vi "Video read with led for 2 part.vi"() -> ()   [LabVIEW 2009]
uses:
  <vilib>/vision/Image Controls.llb/IMAQ Image.ctl
  <vilib>/Instr/_visa.llb/VISA Configure Serial Port (Instr).vi
  <vilib>/Analysis/3filter.llb/Filter Passband Type.ctl
  <vilib>/Analysis/3filter.llb/Butterworth Filter (DBL).vi
  <vilib>/vision/NI_Vision_Development_Module.lvlib
  <vilib>/Analysis/NI_AALBase.lvlib
panel:
  out "cluster":T1
  in  "baud rate (9600)":u32=9600
  in  "VISA resource name":refnum<visa-resource-name>
  out "number":u32
  out "decimal integer string":string
  out "Image Dst Out":T2
  out "Blue Line":T3={"Global Rectangle"=[243, 262, 261, 384], "Contours"=[{"ID"=enum."External", "Type"=2, "Coordinates"=[260, 383, 243, 262]}]} {"Contours"."Type" items=["No Selection", "Point", "Line", "Rectangle", "Oval", "Polygon", "Freehand Region", "Annulus", "Unused2", "Unused3", "Broken Line", "Freehand Line", "Rotated Rectangle"]}
  out "Red Line":T3={"Global Rectangle"=[168, 264, 180, 378], "Contours"=[{"ID"=enum."External", "Type"=2, "Coordinates"=[168, 377, 179, 264]}]} {"Contours"."Type" items=["No Selection", "Point", "Line", "Rectangle", "Oval", "Polygon", "Freehand Region", "Annulus", "Unused2", "Unused3", "Broken Line", "Freehand Line", "Rotated Rectangle"]}
  in  "low  2":dbl=0.12500000000000006 format="%0.4f"
  in  "high 2":dbl=60.0 format="%0.2f"
  in  "sampling 2":dbl=1.0 format="%0.2f"
  out "LED BLUE":bool
  out "Waveform BLUE":dbl[](graph)
  in  "playtime":dbl=30.0
  out "Frame Number":i32
  in  "Frame Start":i32=2400
  out "LED RED":bool
  in  "low":dbl=0.12500000000000006 format="%0.4f"
  out "Waveform RED":dbl[](graph)
  in  "high":dbl=60.0 format="%0.2f"
  in  "sampling":dbl=1.0 format="%0.2f"
  out "Image":T2(plugin-control)
  in  "stop":bool
  in  "AVI Path":path
  # "RED"
  # "BLUE"
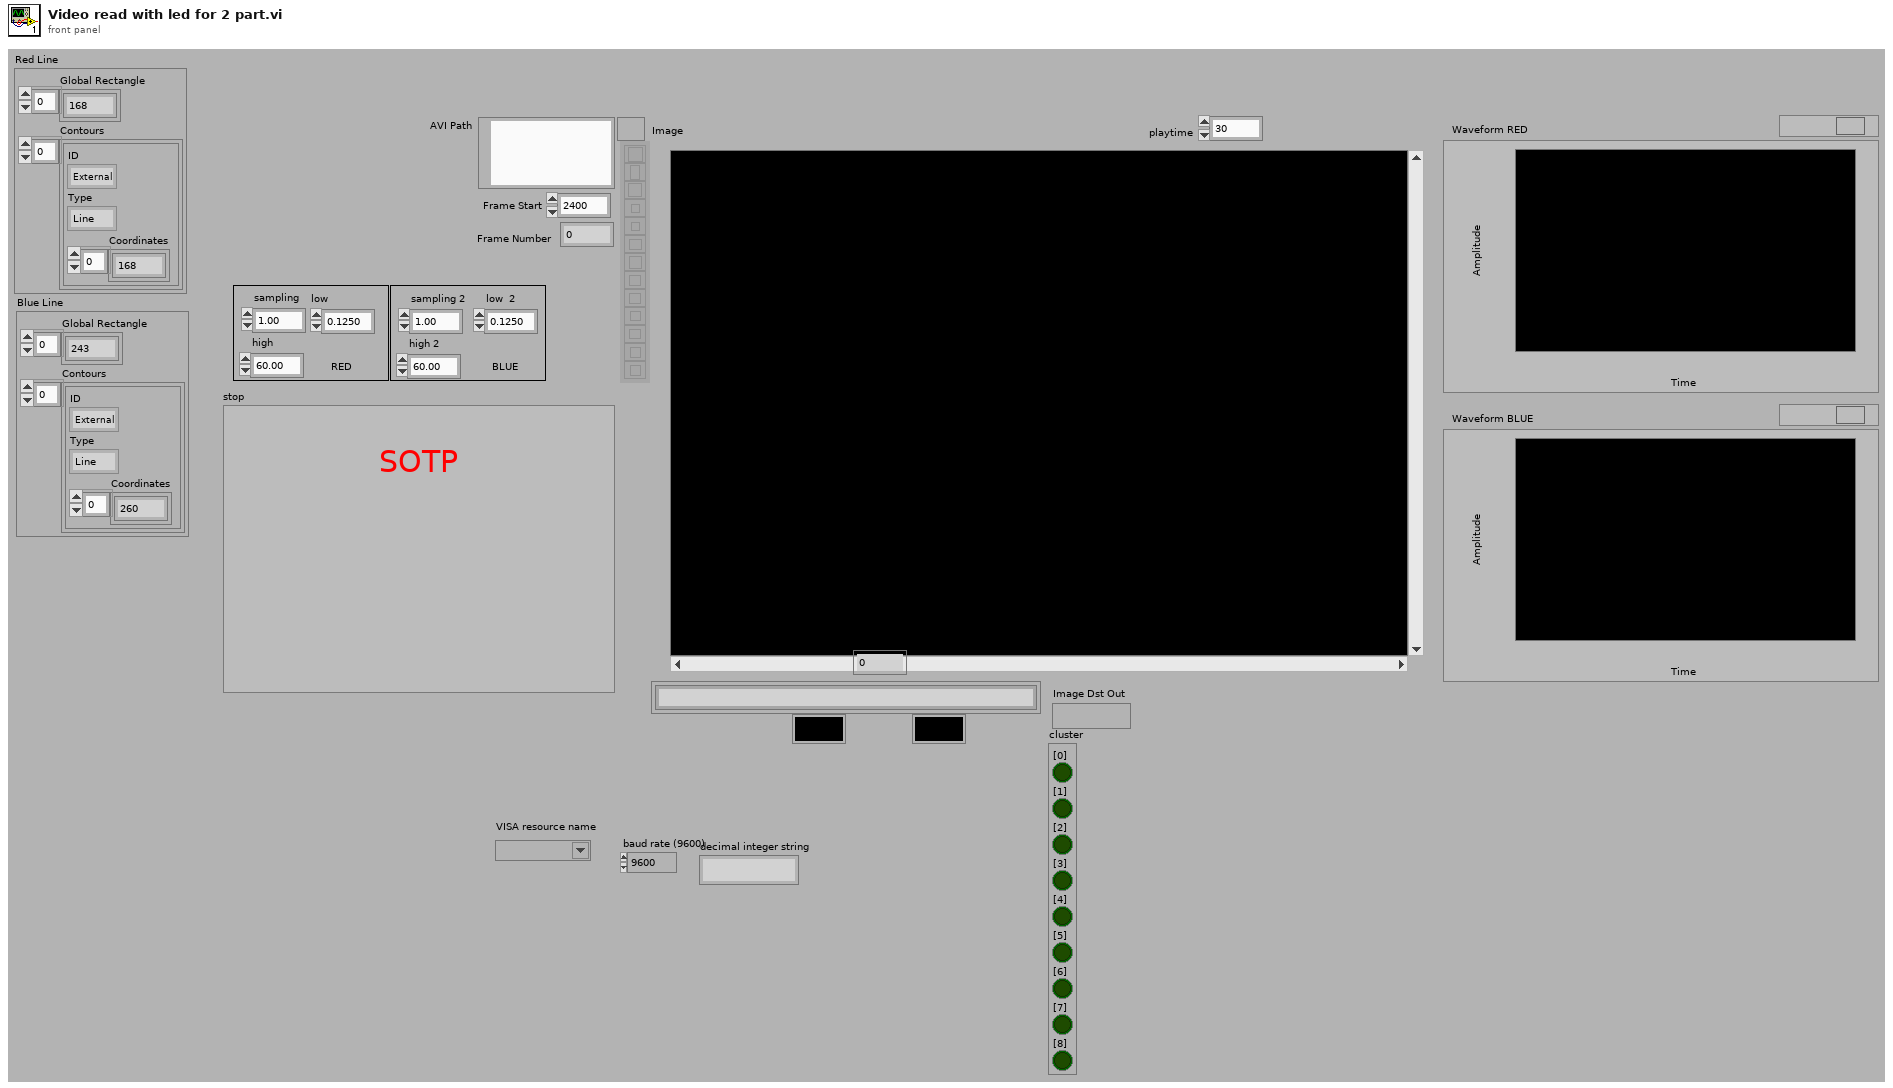
[diagram p1: front panel]
types:
  T1 = cluster{"[0]":bool, "[1]":bool, "[2]":bool, "[3]":bool, "[4]":bool, "[5]":bool, "[6]":bool, "[7]":bool, "[8]":bool}
  T2 = typedef "IMAQ Image.ctl" = refnum<image>
  T3 = cluster{"Global Rectangle":i32[], "Contours":cluster{"ID":enum32{"External", "Internal"}, "Type":u32, "Coordinates":i32[]}[]}
  T4 = typedef "NI_AALBase.lvlib/Filter Passband Type.ctl" = enum32{"Lowpass", "Highpass", "Bandpass", "Bandstop"}
  T5 = cluster{"Left":i32, "Top":i32, "Right":i32, "Bottom":i32}
  T6 = typedef "Image Type" = u32
  T7 = typedef "AviRefnum.ctl" = refnum<k1>
  T8 = cluster{"ID":enum32{"External", "Internal"}, "Type":u32, "Coordinates":i32[]}[]
  T9 = cluster{"ID":enum32{"External", "Internal"}, "Type":u32, "Coordinates":i32[]}
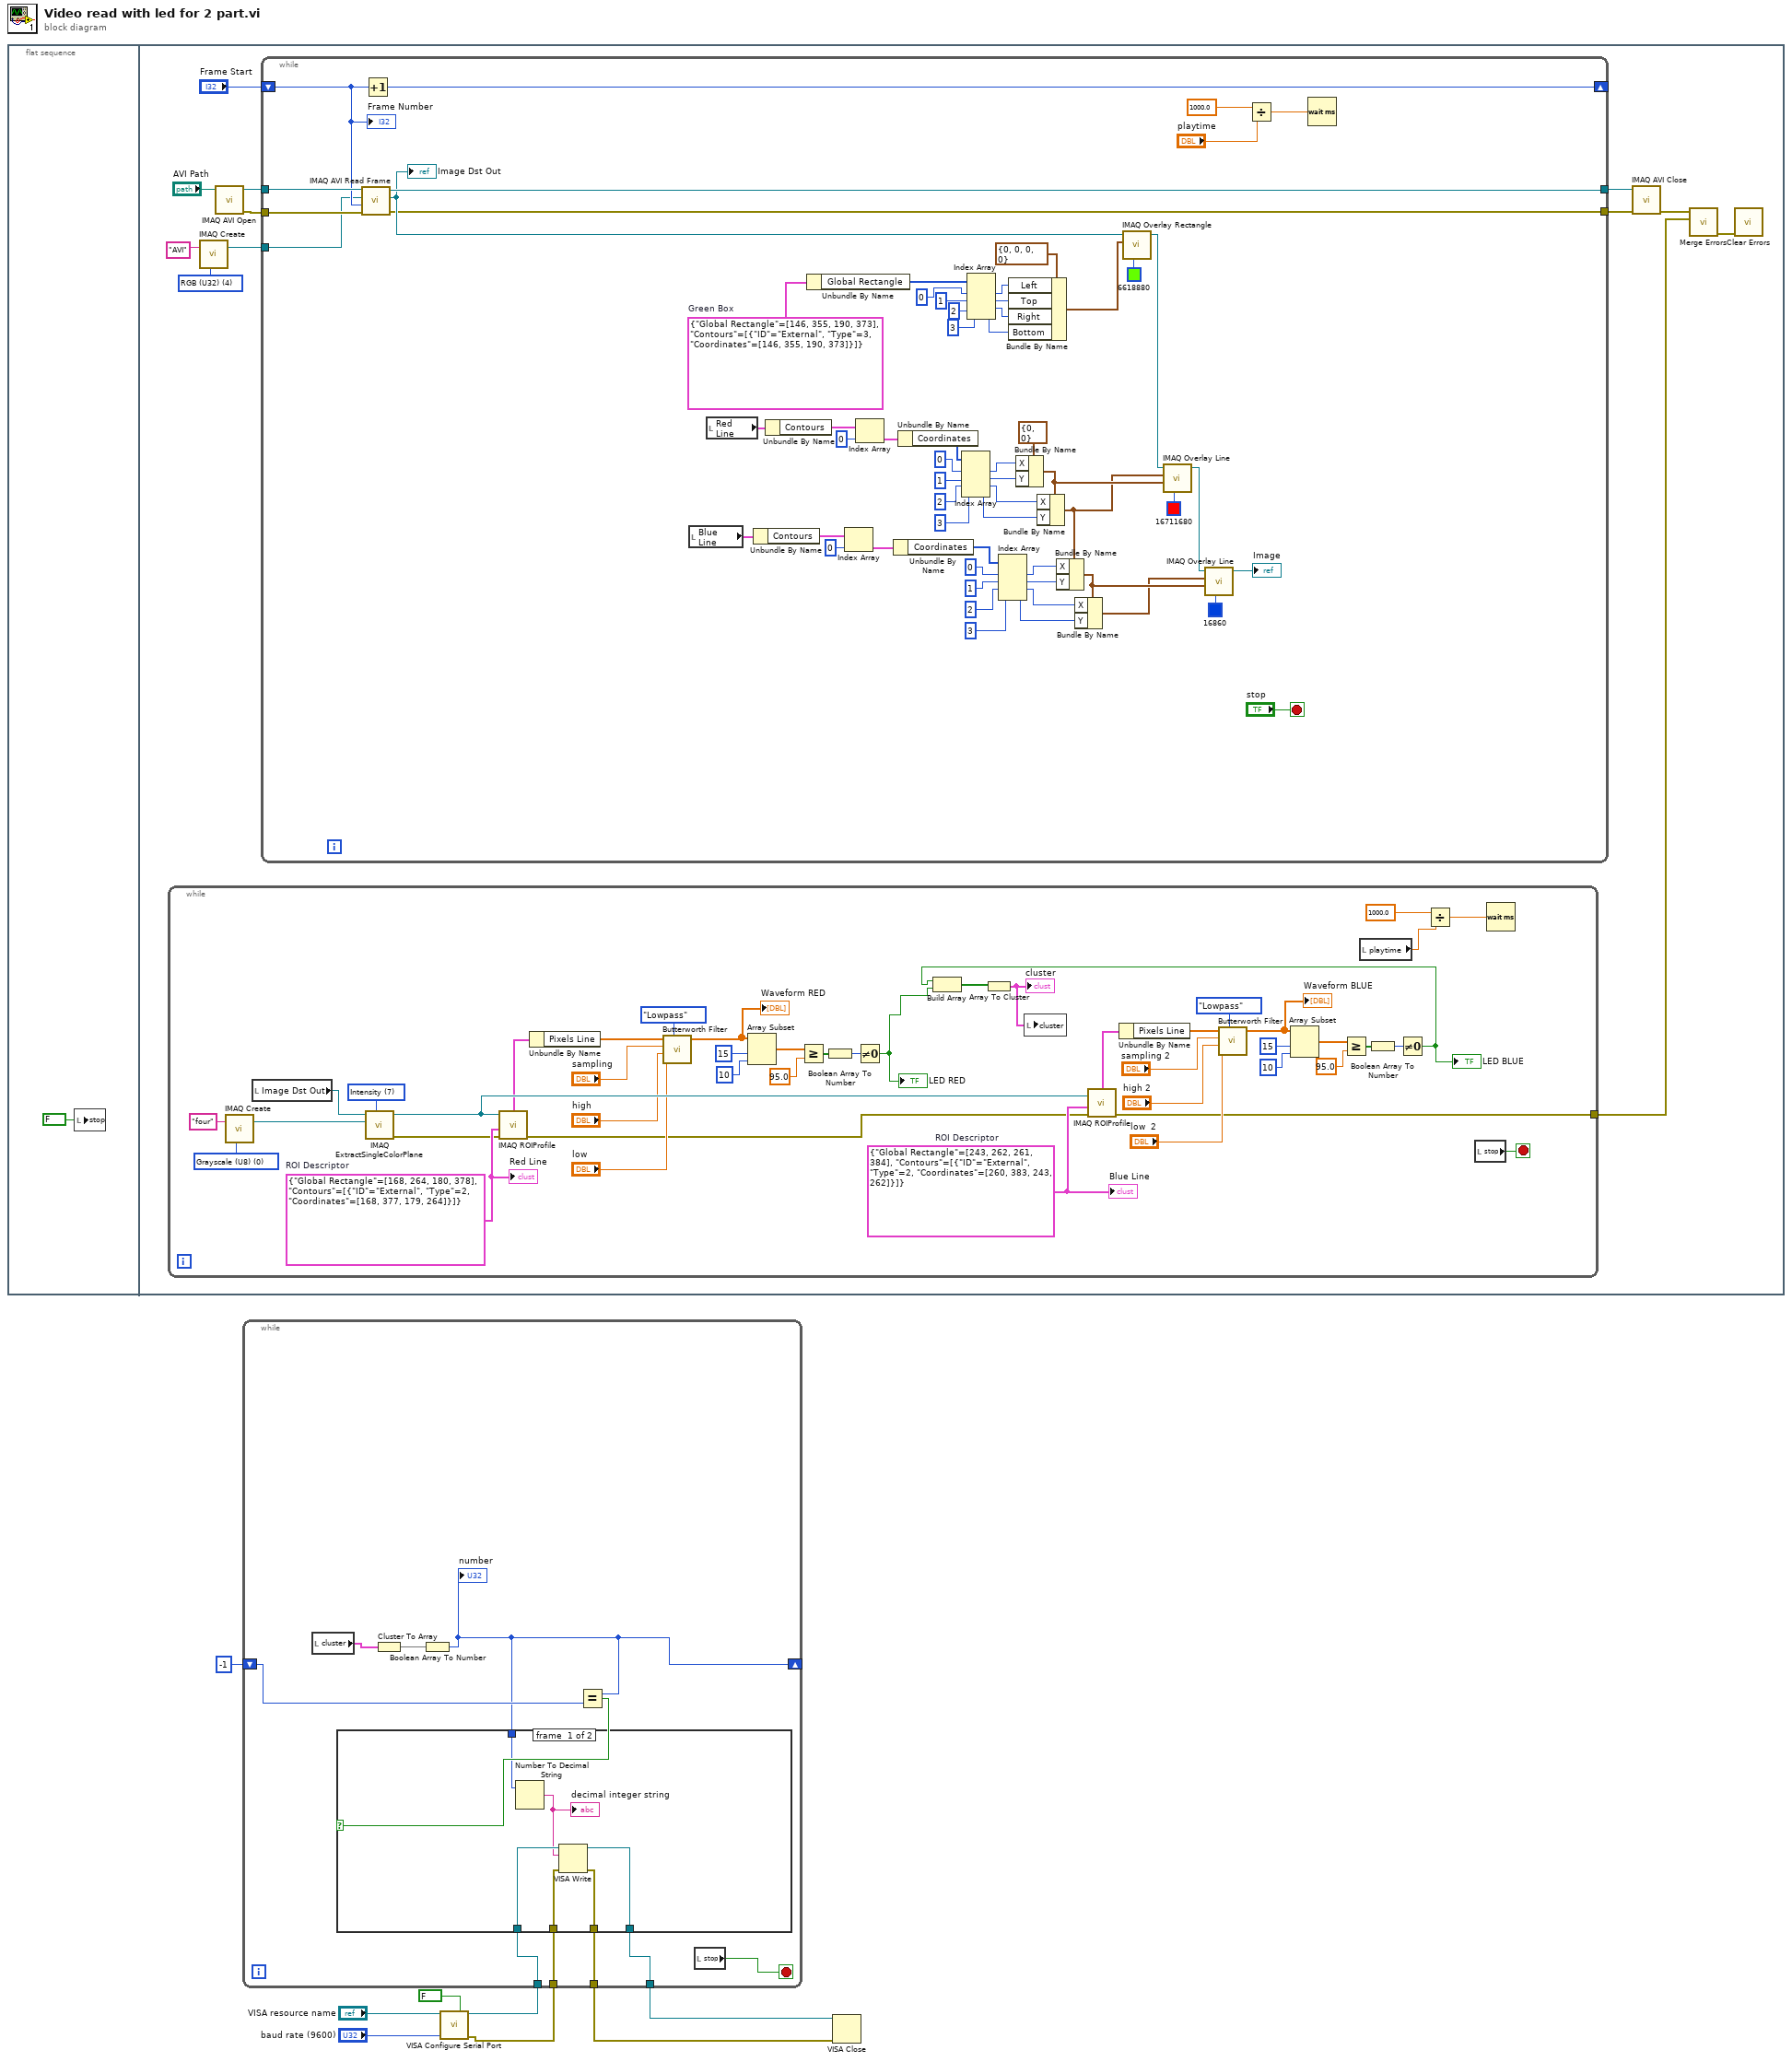
[diagram p0: block diagram]
diagram:
  n1 = flat-sequence {
    frame #0 {
      n2 = local write "stop"(FALSE ("stop")) -> ()
    }
    frame #1 {
      w12 = T6 4 items=["Grayscale (U8)", "Grayscale (I16)", "Grayscale (SGL)", "Complex (CSG)", "RGB (U32)", "HSL (U32)", "RGB (U64)", "Grayscale (U16)"] ("Image Type")
      n3 = while {
        tunnel: [w29] -> w15
        stop <- w64 stop-if-true
        w28 = T6 0 items=["Grayscale (U8)", "Grayscale (I16)", "Grayscale (SGL)", "Complex (CSG)", "RGB (U32)", "HSL (U32)", "RGB (U64)", "Grayscale (U16)"] ("Image Type")
        w62 = T3 {"Global Rectangle"=[243, 262, 261, 384], "Contours"=[{"ID"=enum."External", "Type"=2, "Coordinates"=[260, 383, 243, 262]}]}  # ROI Descriptor
        w63 = T3 {"Global Rectangle"=[168, 264, 180, 378], "Contours"=[{"ID"=enum."External", "Type"=2, "Coordinates"=[168, 377, 179, 264]}]}  # ROI Descriptor
        w66 = 7 items=["Red", "Green", "Blue", "Hue", "Saturation", "Luminance", "Value", "Intensity"] ("Color Plane")
        n4 = call "IMAQ Create"("Image Name"="four", "Image Type"=w28) -> ("New Image"=w26:T2)  [unwired: 3 in, 1 out]
        n5 = local read "Image Dst Out"() -> (w31:T2)
        n6 = call "IMAQ ExtractSingleColorPlane"("Color Plane"=w66, "Image Dst"=w26, "Image Src"=w31) -> ("error out"=w30:errorcluster, "Image Dst Out"=w65:T2)  [unwired: 1 in, 6 out]
        n7 = call "IMAQ ROIProfile"("error in (no error)"=w30, "ROI Descriptor"=w63, "Image"=w65) -> ("error out"=w32:errorcluster, "ROI Graph"=w60:cluster{"x0":sgl, "dx":sgl, "Pixels Line":sgl[]})  [unwired: 4 out]
        n8 = Unbundle By Name(w60) -> ("Pixels Line"=w59:sgl[])
        n9 = call-poly <vilib>:"Butterworth Filter.vi"("filter type"=Filter_Passband_Type."Lowpass", "low cutoff freq: fl"="low", "high cutoff freq: fh"="high", "sampling freq: fs"="sampling", "X"=w59) -> ("Filtered X"=w55:dbl[])  [unwired: 3 in, 1 out]
        "Waveform RED" <- w55
        n10 = Array Subset(array=w55, index=15, length=10) -> (w52:dbl[])
        n11 = Greater Or Equal?(x=w52, y=95.0) -> (x >= y?=w50:bool[])
        n12 = Boolean Array To Number(Boolean array=w50) -> (number=w47:u32)
        n13 = Not Equal To 0?(x=w47) -> (x != 0?=w22:bool)
        "LED RED" <- w22
        n14 = call "IMAQ ROIProfile"("error in (no error)"=w32, "ROI Descriptor"=w62, "Image"=w65) -> ("error out"=w29:errorcluster, "ROI Graph"=w35:cluster{"x0":sgl, "dx":sgl, "Pixels Line":sgl[]})  [unwired: 4 out]
        n15 = Unbundle By Name(w35) -> ("Pixels Line"=w38:sgl[])
        n16 = call-poly <vilib>:"Butterworth Filter.vi"("filter type"=Filter_Passband_Type."Lowpass", "low cutoff freq: fl"="low  2", "high cutoff freq: fh"="high 2", "sampling freq: fs"="sampling 2", "X"=w38) -> ("Filtered X"=w34:dbl[])  [unwired: 3 in, 1 out]
        "Waveform BLUE" <- w34
        n17 = Array Subset(array=w34, index=15, length=10) -> (w43:dbl[])
        n18 = Greater Or Equal?(x=w43, y=95.0) -> (x >= y?=w41:bool[])
        n19 = local read "playtime"() -> (w46:dbl)
        n20 = Boolean Array To Number(Boolean array=w41) -> (number=w40:u32)
        n21 = Not Equal To 0?(x=w40) -> (x != 0?=w23:bool)
        "LED BLUE" <- w23
        n22 = Build Array(w23, w22) -> (w25:bool[])
        n23 = Array To Cluster(array=w25) -> (cluster=w24:T1)
        "cluster" <- w24
        n24 = local write "cluster"(w24) -> ()
        n25 = Divide(x=1000.0, y=w46) -> (x/y=w49:dbl)
        n26 = local read "stop"() -> (w64:bool)
        n27 = Wait (ms)(milliseconds to wait=w49) -> ()  [unwired: 1 out]
        "Red Line" <- w63
        "Blue Line" <- w62
      }
      n28 = call "IMAQ Create"("Image Name"="AVI", "Image Type"=w12) -> ("New Image"=w10:T2)  [unwired: 3 in, 1 out]
      n29 = call "IMAQ AVI Open"("AVI Path"="AVI Path") -> ("error out"=w18:errorcluster, "Avi Refnum"=w19:T7)  [unwired: 9 in]
      n30 = while {
        tunnel: w19 -> [w127]
        tunnel: w18 -> [w72]
        tunnel: [w126] -> w20
        shift-right: [w121] -> _
        shift-left: "Frame Start" -> [w120]
        tunnel: [w68] -> w13
        tunnel: w10 -> [w67]
        stop <- "stop" stop-if-true
        w119 = T3 {"Global Rectangle"=[146, 355, 190, 373], "Contours"=[{"ID"=enum."External", "Type"=3, "Coordinates"=[146, 355, 190, 373]}]}  # Green Box
        n31 = call "IMAQ AVI Read Frame"("error in (no error)"=w72, "Frame Number"=w120, "Image"=w67, "Avi Refnum"=w127) -> ("error out"=w68:errorcluster, "Image Out"=w69:T2, "Avi Refnum (duplicate)"=w126:T7)  [unwired: 4 in, 1 out]
        "Image Dst Out" <- w69
        n32 = Increment(x=w120) -> (x+1=w121:i32)
        n33 = local read "Blue Line"() -> (w71:T3)
        n34 = local read "Red Line"() -> (w70:T3)
        n35 = Unbundle By Name(w71) -> ("Contours"=w86:T8)
        n36 = Unbundle By Name(w70) -> ("Contours"=w101:T8)
        n37 = Unbundle By Name(w119) -> ("Global Rectangle"=w115:i32[])
        n38 = Index Array(array=w86, index=0) -> (element=w85:T9)
        n39 = Index Array(array=w101, index=0) -> (element=w103:T9)
        n40 = Unbundle By Name(w85) -> ("Coordinates"=w84:i32[])
        n41 = Unbundle By Name(w103) -> ("Coordinates"=w104:i32[])
        n42 = Index Array(array=w104, index #1=0 ("index"), index #2=1 ("index"), index #3=2 ("index"), index #4=3 ("index")) -> (element #1=w96:i32, element #2=w97:i32, element #3=w98:i32, element #4=w99:i32)
        n43 = Index Array(array=w115, index #1=0 ("index"), index #2=1 ("index"), index #3=2 ("index"), index #4=3 ("index")) -> (element #1=w114:i32, element #2=w113:i32, element #3=w112:i32, element #4=w111:i32)
        n44 = Index Array(array=w84, index #1=0 ("index"), index #2=1 ("index"), index #3=2 ("index"), index #4=3 ("index")) -> (element #1=w83:i32, element #2=w89:i32, element #3=w88:i32, element #4=w87:i32)
        n45 = Bundle By Name(cluster=T5 {"Left"=0, "Top"=0, "Right"=0, "Bottom"=0} ("Rectangle"), "Left"=w114, "Top"=w113, "Right"=w112, "Bottom"=w111) -> (w117:T5)
        n46 = Bundle By Name(cluster=cluster{"X":i32, "Y":i32} {"X"=0, "Y"=0} ("End Point"), "X"=w96, "Y"=w97) -> (w105:cluster{"X":i32, "Y":i32})
        n47 = Bundle By Name(cluster=w105, "X"=w98, "Y"=w99) -> (w75:cluster{"X":i32, "Y":i32})
        n48 = Bundle By Name(cluster=w75, "X"=w83, "Y"=w89) -> (w90:cluster{"X":i32, "Y":i32})
        n49 = Bundle By Name(cluster=w90, "X"=w88, "Y"=w87) -> (w81:cluster{"X":i32, "Y":i32})
        n50 = call "IMAQ Overlay Rectangle"("Color"=u32 6618880, "Rectangle"=w117, "Image"=w69) -> ("Image Out"=w91:T2)  [unwired: 7 in, 1 out]
        n51 = call "IMAQ Overlay Line"("Color"=u32 16711680, "End Point"=w105, "Start Point"=w75, "Image"=w91) -> ("Image Out"=w80:T2)  [unwired: 6 in, 1 out]
        n52 = call "IMAQ Overlay Line"("Color"=u32 16860, "End Point"=w90, "Start Point"=w81, "Image"=w80) -> ("Image Out"=→"Image":T2)  [unwired: 6 in, 1 out]
        n53 = Divide(x=1000.0, y="playtime") -> (x/y=w124:dbl)
        n54 = Wait (ms)(milliseconds to wait=w124) -> ()  [unwired: 1 out]
        "Frame Number" <- w120
      }
      n55 = call "IMAQ AVI Close"("error in (no error)"=w13, "Avi Refnum"=w20) -> ("error out"=w16:errorcluster)  [unwired: 9 in]
      n56 = call <vilib>:"Merge Errors.vi"("error in 2 (no error)"=w15, "error in 1 (no error)"=w16) -> ("error out"=w14:errorcluster)  [unwired: 5 in]
      n57 = call <vilib>:"Clear Errors.vi"("error in (no error)"=w14) -> ()  [unwired: 6 in, 1 out]
    }
  }
  n58 = call-poly "VISA Configure Serial Port"("VISA resource name"="VISA resource name", "Enable Termination\nChar (T)"=FALSE ("Enable Termination\nChar (T)"), "baud rate (9600)"="baud rate (9600)") -> ("VISA resource name out"=w7:refnum<visa-resource-name>, "error out"=w2:errorcluster)  [unwired: 11 in]
  n59 = while {
    shift-right: [w131] -> _
    shift-left: -1 -> [w137]
    tunnel: w7 -> [w135]
    tunnel: [w134] -> w6
    tunnel: w2 -> [w133]
    tunnel: [w132] -> w1
    stop <- w128 stop-if-true
    n60 = local read "cluster"() -> (w129:T1)
    n61 = Cluster To Array(cluster=w129) -> (array=w130:bool[])
    n62 = Boolean Array To Number(Boolean array=w130) -> (number=w131:u32)
    "number" <- w131
    n63 = Equal?(x=w131, y=w137) -> (x = y?=w136:bool)
    n64 = case shown="False" w136 {
      tunnel: w135 -> [w143 w145]
      tunnel: [w142 w145] -> w134
      tunnel: w131 -> [w140 _]
      tunnel: w133 -> [w139 w144]
      tunnel: [w138 w144] -> w132
      frame #0 {
        n65 = Number To Decimal String(number=w140) -> (decimal integer string=w141:string)  [unwired: 1 in]
        "decimal integer string" <- w141
        n66 = VISA Write(VISA resource name=w143, write buffer=w141, error in (no error)=w139) -> (VISA resource name out=w142:refnum<visa-resource-name>, error out=w138:errorcluster)  [unwired: 1 out]
      }
      frame #1 {
      }
    }
    n67 = local read "stop"() -> (w128:bool)
  }
  n68 = VISA Close(VISA resource name=w6, error in (no error)=w1) -> ()  [unwired: 1 out]
